vi "MoveMI_in_vert.vi"(8 "error in (no error)":errorcluster) -> (0 "error out":errorcluster, 3 "in range is True":bool)   [LabVIEW 2020]
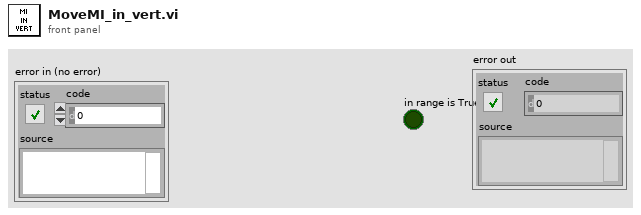
[diagram p1: front panel]
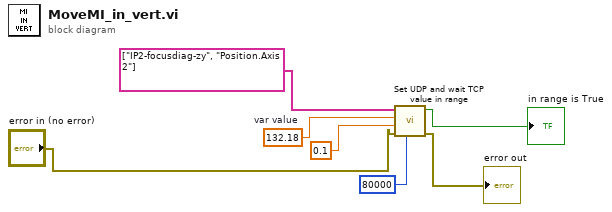
[diagram p0: block diagram]
diagram:
  w6 = 132.18  # var value
  n1 = call "Set UDP and wait TCP value in range.vi"("timeout"=80000 ("slow timeout ms (3000)"), "error in (no error)"="error in (no error)", "tolerance"=0.1, "set value"=w6, "device and variable"=string[] ["IP2-focusdiag-zy", "Position.Axis 2"] ("dev variable alias Motors X")) -> ("error out"=→"error out":errorcluster, "In range is True"=→"in range is True":bool)  [unwired: 5 in]
